vi "MGCC_BlkStart_main.vi"() -> ()   [LabVIEW 2016]
doc: "-----------------------------------------------------------------------------------------------------------------------\nCopyright <2019> <The University of Tennessee at Knoxville and the University of Tennessee Research Foundation>\nThis software is released under BSD-3 \nhttps://opensource.org/licenses/BSD-3-Clause \nAdditional license options available at https://utrf.tennessee.edu/industry/sample-agreements/\n-----------------------------------------------------------------------------------------------------------------------"
uses:
  Finite State Machine/Sub-VIs/MGCC_FntStaMach_gobal.vi
  <vilib>/Utility/error.llb/Error Cluster From Error Code.vi
  <vilib>/ErrorRing/Error Ring.xnode
panel:
  out "Numeric":dbl
  out "Boolean 5":bool
  out "Boolean 4":bool
  out "Boolean 3":bool
  out "Boolean 2":bool
  in  "flag_3=0?":bool
  in  "flag_2=0?":bool
  in  "flag_1=0?":bool
  in  "flag=0?":bool
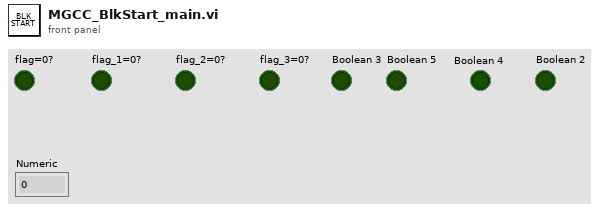
[diagram p1: front panel]
types:
  T1 = cluster{"maxf":dbl, "minf":dbl, "maxV":dbl, "minV":dbl, " PVramp":dbl, "Double":dbl, "Double":dbl, "Double":dbl}
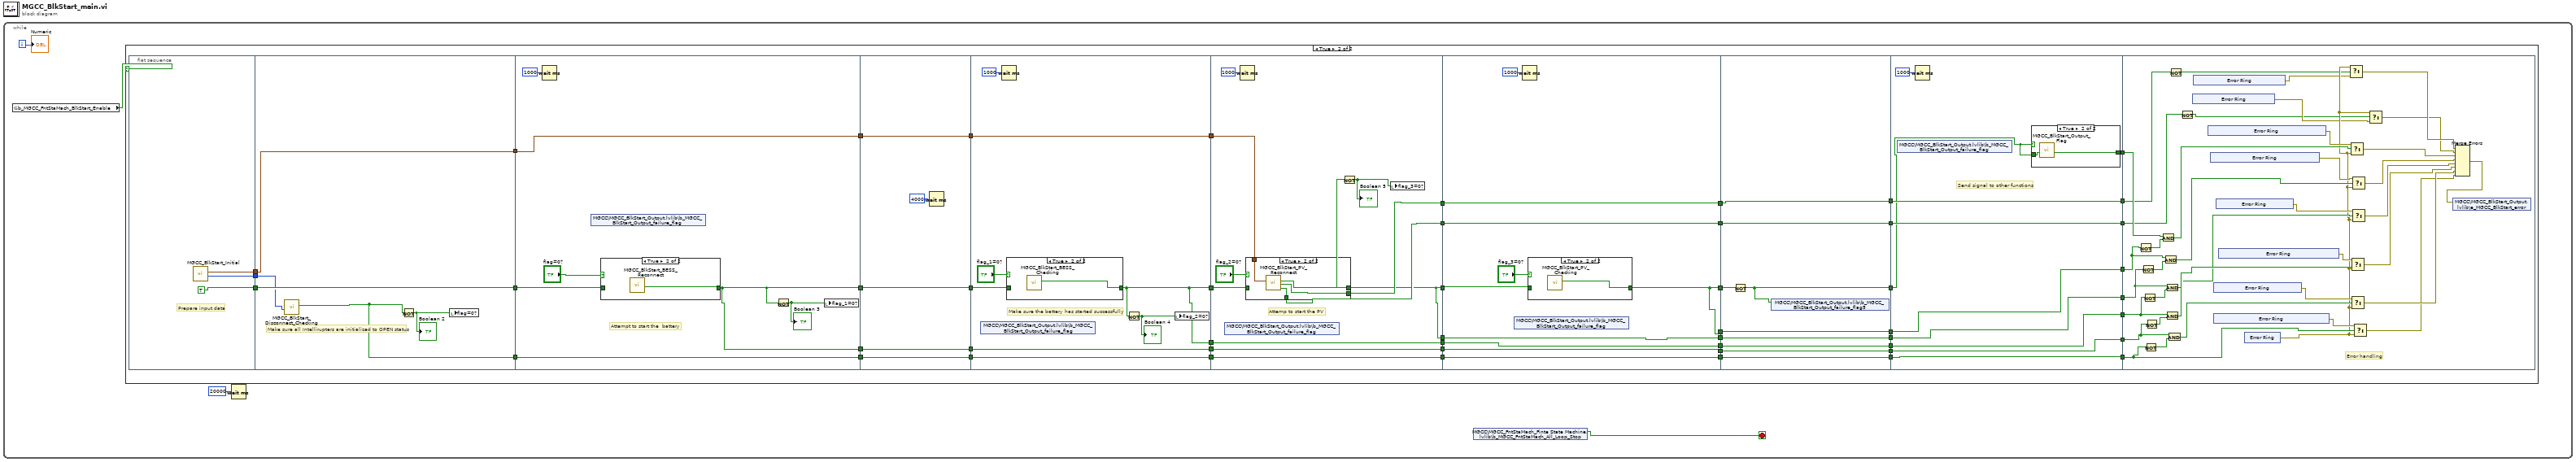
[diagram p0: block diagram]
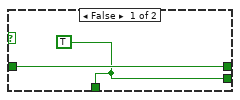
[diagram p5: hidden frame]
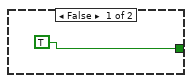
[diagram p7: hidden frame]
diagram:
  n1 = while {
    i -> [w3]
    stop <- w2 stop-if-true
    n2 = global read "MGCC_FntStaMach_gobal.vi" "b_MGCC_FntStaMach_BlkStart_Enable"() -> (w1:bool)
    n3 = case shown="True" w1 {
      frame False {
      }
      frame True {
        n4 = flat-sequence {
          tunnel: [w57] -> w54
          tunnel: [w56] -> w53
          tunnel: [TRUE] -> w51
          tunnel: w54 -> [w60]
          tunnel: w53 -> [w61]
          tunnel: [w62] -> w52
          tunnel: w51 -> [w62]
          tunnel: [w60] -> w46
          tunnel: [w58] -> w42
          tunnel: w52 -> [w67]
          tunnel: [w63] -> w12
          tunnel: w46 -> [w66]
          tunnel: [w66] -> w10
          tunnel: [w63] -> w8
          tunnel: [w65] -> w6
          tunnel: w42 -> [w65]
          tunnel: w12 -> [w76]
          tunnel: [w76] -> w11
          tunnel: w10 -> [w75]
          tunnel: [w75] -> w9
          tunnel: w8 -> [w74]
          tunnel: [w74] -> w7
          tunnel: w6 -> [w73]
          tunnel: [w73] -> w5
          tunnel: w11 -> [w82]
          tunnel: [w77] -> w50
          tunnel: [w81] -> w45
          tunnel: w9 -> [w81]
          tunnel: [w80] -> w44
          tunnel: w7 -> [w80]
          tunnel: [w79] -> w43
          tunnel: w5 -> [w79]
          tunnel: [w77] -> w41
          tunnel: w50 -> [w95]
          tunnel: [w87] -> w49
          tunnel: w45 -> [w94]
          tunnel: w44 -> [w92]
          tunnel: w43 -> [w93]
          tunnel: w41 -> [w91]
          tunnel: [w93] -> w40
          tunnel: [w92] -> w39
          tunnel: [w91] -> w38
          tunnel: [w87] -> w37
          tunnel: [w90] -> w19
          tunnel: [w89] -> w17
          tunnel: w49 -> [w111]
          tunnel: [w106] -> w48
          tunnel: w40 -> [w110]
          tunnel: w39 -> [w109]
          tunnel: w38 -> [w108]
          tunnel: w37 -> [w107]
          tunnel: [w110] -> w36
          tunnel: [w109] -> w35
          tunnel: [w108] -> w34
          tunnel: [w107] -> w33
          tunnel: [w106] -> w32
          tunnel: [w105] -> w20
          tunnel: w19 -> [w105]
          tunnel: [w104] -> w18
          tunnel: w17 -> [w104]
          tunnel: w48 -> [w124]
          tunnel: [w123] -> w47
          tunnel: w36 -> [w122]
          tunnel: w35 -> [w121]
          tunnel: w34 -> [w120]
          tunnel: w33 -> [w119]
          tunnel: w32 -> [w118]
          tunnel: [w122] -> w31
          tunnel: [w121] -> w30
          tunnel: [w120] -> w29
          tunnel: [w119] -> w28
          tunnel: [w118] -> w27
          tunnel: w20 -> [w117]
          tunnel: w18 -> [w116]
          tunnel: [w117] -> w15
          tunnel: [w116] -> w13
          tunnel: w47 -> [w125]
          tunnel: w31 -> [w133]
          tunnel: w30 -> [w132]
          tunnel: w29 -> [w131]
          tunnel: w28 -> [w130]
          tunnel: w27 -> [w129]
          tunnel: [w133] -> w26
          tunnel: [w132] -> w25
          tunnel: [w131] -> w24
          tunnel: [w130] -> w23
          tunnel: [w129] -> w22
          tunnel: [w128] -> w21
          tunnel: [w127] -> w16
          tunnel: w15 -> [w127]
          tunnel: [w126] -> w14
          tunnel: w13 -> [w126]
          tunnel: w26 -> [w174]
          tunnel: w25 -> [w170]
          tunnel: w24 -> [w166]
          tunnel: w23 -> [w164]
          tunnel: w22 -> [w162]
          tunnel: w21 -> [w161]
          tunnel: w16 -> [w141]
          tunnel: w14 -> [w139]
          frame #0 {
            # "Prepare input data"
            n5 = call "MGCC_BlkStart_Initial.vi"() -> ("flag"=w56:i32[], "Output cluster"=w57:T1)  [unwired: 10 in]
          }
          frame #1 {
            # "Make sure all Intellirupters are initialized to OPEN status"
            n6 = call "MGCC_BlkStart_Disconnect_Checking.vi"("flag"=w61) -> ("failure_flag 1"=w58:bool)  [unwired: 10 in]
            n7 = Not(x=w58) -> (.not. x?=w59:bool)
            "Boolean 2" <- w59
            n8 = local write "flag=0?"(w59) -> ()
          }
          frame #2 {
            # "Attempt to start the  battery"
            n9 = Wait (ms)(milliseconds to wait=1000) -> ()  [unwired: 1 out]
            n10 = shared-variable "MGCC\\MGCC_BlkStart_Output.lvlib\\b_MGCC_BlkStart_Output_failure_flag"() -> ()  [unwired: 1 in, 2 out]
            n11 = case shown="True" "flag=0?" {
              tunnel: w67 -> [w70 _]
              tunnel: [w70 w71] -> w63
              frame False {
              }
              frame True {
                n12 = call "MGCC_BlkStart_BESS_Reconnect.vi"() -> ("failure_flag 2"=w71:bool)  [unwired: 11 in]
              }
            }
            n13 = Not(x=w63) -> (.not. x?=w64:bool)
            "Boolean 3" <- w64
            n14 = local write "flag_1=0?"(w64) -> ()
          }
          frame #3 {
            n15 = Wait (ms)(milliseconds to wait=4000) -> ()  [unwired: 1 out]
          }
          frame #4 {
            # "Make sure the battery has started successfully"
            n16 = shared-variable "MGCC\\MGCC_BlkStart_Output.lvlib\\b_MGCC_BlkStart_Output_failure_flag"() -> ()  [unwired: 1 in, 2 out]
            n17 = Wait (ms)(milliseconds to wait=1000) -> ()  [unwired: 1 out]
            n18 = case shown="True" "flag_1=0?" {
              tunnel: w82 -> [w85 _]
              tunnel: [w85 w86] -> w77
              frame False {
              }
              frame True {
                n19 = call "MGCC_BlkStart_BESS_Checking.vi"() -> ("failure_flag 3"=w86:bool)  [unwired: 11 in]
              }
            }
            n20 = Not(x=w77) -> (.not. x?=w78:bool)
            "Boolean 4" <- w78
            n21 = local write "flag_2=0?"(w78) -> ()
          }
          frame #5 {
            # "Attemp to start the PV"
            n22 = shared-variable "MGCC\\MGCC_BlkStart_Output.lvlib\\b_MGCC_BlkStart_Output_failure_flag"() -> ()  [unwired: 1 in, 2 out]
            n23 = Wait (ms)(milliseconds to wait=1000) -> ()  [unwired: 1 out]
            n24 = case shown="True" "flag_2=0?" {
              tunnel: [w99 w103] -> w87
              tunnel: w95 -> [w99 _]
              tunnel: w94 -> [_ w102]
              tunnel: [w98 w101] -> w90
              tunnel: [w98 w100] -> w89
              frame False {
                w98 = TRUE
              }
              frame True {
                n25 = call "MGCC_BlkStart_PV_Reconnect.vi"("Input cluster"=w102) -> ("Vlim"=w100:bool, "flim"=w101:bool, "failure_flag 3"=w103:bool)  [unwired: 8 in]
              }
            }
            n26 = Not(x=w87) -> (.not. x?=w88:bool)
            "Boolean 5" <- w88
            n27 = local write "flag_3=0?"(w88) -> ()
          }
          frame #6 {
            # "Make sure the PV has started successfully"
            n28 = shared-variable "MGCC\\MGCC_BlkStart_Output.lvlib\\b_MGCC_BlkStart_Output_failure_flag"() -> ()  [unwired: 1 in, 2 out]
            n29 = Wait (ms)(milliseconds to wait=1000) -> ()  [unwired: 1 out]
            n30 = case shown="True" "flag_3=0?" {
              tunnel: [w114 w115] -> w106
              tunnel: w111 -> [w114 _]
              frame False {
              }
              frame True {
                n31 = call "MGCC_BlkStart_PV_Checking.vi"() -> ("failure_flag 4"=w115:bool)  [unwired: 11 in]
              }
            }
          }
          frame #7 {
            n32 = Not(x=w124) -> (.not. x?=w123:bool)
            n33 = shared-variable "MGCC\\MGCC_BlkStart_Output.lvlib\\b_MGCC_BlkStart_Output_failure_flag5"(w123) -> ()  [unwired: 1 in, 1 out]
          }
          frame #8 {
            # "Send signal to other functions"
            n34 = shared-variable "MGCC\\MGCC_BlkStart_Output.lvlib\\b_MGCC_BlkStart_Output_failure_flag"() -> ()  [unwired: 1 in, 2 out]
            n35 = Wait (ms)(milliseconds to wait=1000) -> ()  [unwired: 1 out]
            n36 = case shown="True" w125 {
              tunnel: [TRUE w137] -> w128
              tunnel: w125 -> [_ w136]
              frame False {
              }
              frame True {
                n37 = call "MGCC_BlkStart_Output_Flag.vi"("BKS_falilure"=w136) -> ("Boolean 3"=w137:bool)  [unwired: 10 in]
              }
            }
          }
          frame #9 {
            # "Error handling"
            n38 = Not(x=w162) -> (.not. x?=w160:bool)
            n39 = Not(x=w164) -> (.not. x?=w163:bool)
            n40 = Not(x=w166) -> (.not. x?=w165:bool)
            n41 = Not(x=w174) -> (.not. x?=w173:bool)
            n42 = Not(x=w170) -> (.not. x?=w169:bool)
            n43 = And(x=w161, y=w160) -> (x .and. y?=w159:bool)
            n44 = And(x=w162, y=w163) -> (x .and. y?=w158:bool)
            n45 = And(x=w164, y=w165) -> (x .and. y?=w157:bool)
            n46 = And(x=w166, y=w169) -> (x .and. y?=w168:bool)
            n47 = And(x=w170, y=w173) -> (x .and. y?=w172:bool)
            n48 = Not(x=w141) -> (.not. x?=w140:bool)
            n49 = Not(x=w139) -> (.not. x?=w138:bool)
            n50 = xnode "Error Ring"() -> ("error out"=w151:errorcluster)
            n51 = xnode "Error Ring"() -> ("error out"=w152:errorcluster)
            n52 = xnode "Error Ring"() -> ("error out"=w155:errorcluster)
            n53 = xnode "Error Ring"() -> ("error out"=w154:errorcluster)
            n54 = xnode "Error Ring"() -> ("error out"=w171:errorcluster)
            n55 = xnode "Error Ring"() -> ("error out"=w175:errorcluster)
            n56 = xnode "Error Ring"() -> ("error out"=w156:errorcluster)
            n57 = xnode "Error Ring"() -> ("error out"=w167:errorcluster)
            n58 = xnode "Error Ring"() -> ("error out"=w153:errorcluster)
            n59 = Select(t=w153, s=w140, f=w152) -> (s? t:f=w150:errorcluster)
            n60 = Select(t=w155, s=w159, f=w153) -> (s? t:f=w148:errorcluster)
            n61 = Select(t=w167, s=w168, f=w153) -> (s? t:f=w145:errorcluster)
            n62 = Select(t=w171, s=w172, f=w153) -> (s? t:f=w144:errorcluster)
            n63 = Select(t=w154, s=w158, f=w153) -> (s? t:f=w147:errorcluster)
            n64 = Select(t=w156, s=w157, f=w153) -> (s? t:f=w146:errorcluster)
            n65 = Select(t=w175, s=w174, f=w153) -> (s? t:f=w143:errorcluster)
            n66 = Select(t=w153, s=w138, f=w151) -> (s? t:f=w149:errorcluster)
            n67 = Merge Errors(w150, w149, w148, w147, w146, w145, w144, w143) -> (w142:errorcluster)
            n68 = shared-variable "MGCC\\MGCC_BlkStart_Output.lvlib\\e_MGCC_BlkStart_error"(w142) -> ()  [unwired: 1 in, 1 out]
          }
        }
      }
    }
    n69 = Wait (ms)(milliseconds to wait=20000) -> ()  [unwired: 1 out]
    n70 = shared-variable "MGCC\\MGCC_FntStaMach_Finte State Machine.lvlib\\b_MGCC_FntStaMach_All_Loop_Stop"() -> (w2:bool)  [unwired: 1 in, 1 out]
    "Numeric" <- w3
  }
